vi "FGV Span.vi"(6 "Aktion":T1, 8 "Aktiv":bool, 9 "Offset":sgl[](array[numeric]), 11 "Span":sgl[](array[numeric])) -> (0 "Aktiv":bool, 1 "Offset":sgl[](array[numeric]), 2 "Aktualisiert":bool, 3 "Span":sgl[](array[numeric]))   [LabVIEW 2020, in "FT-IR.lvlib" / "Spanfaktor.lvlib"]
uses:
  Spanfaktor.lvlib
  Aktion FGV Span.ctl
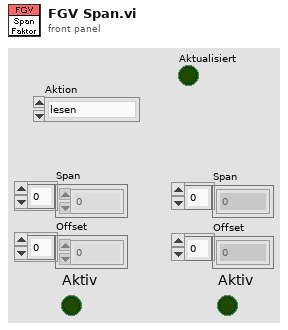
[diagram p1: front panel]
types:
  T1 = typedef "FT-IR.lvlib/Spanfaktor.lvlib/Aktion FGV Span.ctl" = enum16{"lesen", "Span", "Seite aktiv", "Offset", "FGV aktualisiert", "Aktualisierung aufheben"}
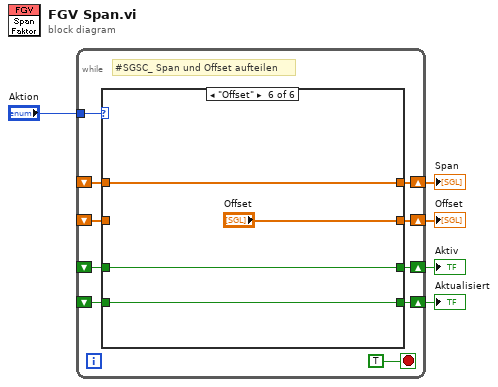
[diagram p0: block diagram]
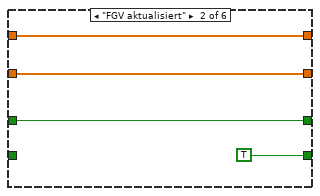
[diagram p3: hidden frame]
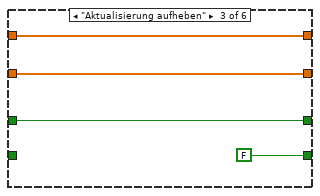
[diagram p4: hidden frame]
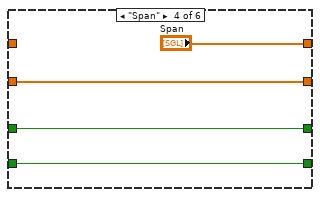
[diagram p5: hidden frame]
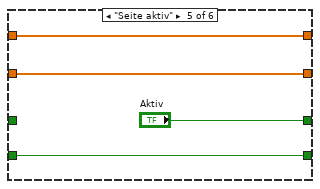
[diagram p6: hidden frame]
diagram:
  n1 = while {
    tunnel: "Aktion" -> [w14]
    shift-right: [w12] -> w3
    shift-left: _ -> [w10]
    shift-right: [w13] -> w4
    shift-left: _ -> [w11]
    shift-right: [w9] -> w2
    shift-left: _ -> [w8]
    shift-right: [w7] -> w1
    shift-left: _ -> [w6]
    stop <- TRUE stop-if-true
    # "#SGSC_ Span und Offset aufteilen"
    n2 = case shown="\"Offset\"" w14 {
      tunnel: [w19 w23 w27 "Span" w35 w39] -> w13
      tunnel: [w18 w22 w26 w29 w34 "Offset"] -> w12
      tunnel: w11 -> [w19 w23 w27 _ w35 w39]
      tunnel: w10 -> [w18 w22 w26 w29 w34 _]
      tunnel: [w17 w21 w25 w30 "Aktiv" w38] -> w9
      tunnel: w8 -> [w17 w21 w25 w30 _ w38]
      tunnel: [w16 TRUE FALSE w28 w32 w36] -> w7
      tunnel: w6 -> [w16 _ _ w28 w32 w36]
      frame "lesen", Default {
      }
      frame "FGV aktualisiert" {
      }
      frame "Aktualisierung aufheben" {
      }
      frame "Span" {
      }
      frame "Seite aktiv" {
      }
      frame "Offset" {
      }
    }
  }
  "Span" <- w4
  "Offset" <- w3
  "Aktiv" <- w2
  "Aktualisiert" <- w1
